vi "Devide_Str_wDel.vi"(2 "Del":string, 3 "Conc String":string) -> (1 "Array":string[](array[string]))   [LabVIEW 2009]
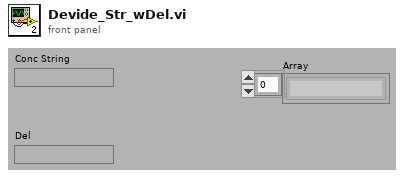
[diagram p1: front panel]
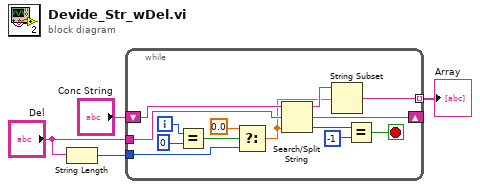
[diagram p0: block diagram]
diagram:
  n1 = String Length(string="Del") -> (length=w1:i32)
  n2 = while {
    tunnel: "Del" -> [w17]
    shift-right: [w16] -> _
    shift-left: "Conc String" -> [w18]
    tunnel: [w7] -> w3 mode=indexing
    tunnel: w1 -> [w6]
    i -> [w15]
    stop <- w9 stop-if-true
    n3 = Equal?(x=w15, y=0) -> (x = y?=w13:bool)
    n4 = Select(t=0.0, s=w13, f=w6) -> (s? t:f=w5:dbl)
    n5 = Search/Split String(string=w18, search string/char (-)=w17, offset (0)=w5) -> (substring before match=w8:string, match + rest of string=w16:string, offset of match=w11:i32)
    n6 = String Subset(string=w8, offset (0)=w5) -> (substring=w7:string)  [unwired: 1 in]
    n7 = Equal?(x=w11, y=-1) -> (x = y?=w9:bool)
  }
  "Array" <- w3
